vi "source_config.vi"(4 "Multimeter":refnum<visa-resource-name>="GPIB0::7::INSTR", 7 "Sourcemeter":refnum<visa-resource-name>="GPIB0::5::INSTR", 8 "error in (no error)":errorcluster, 9 "Compliance  Level (0.1)":dbl=0.1 step=0.001, 10 "Pas":dbl, 11 "Max":dbl) -> (0 "I(OUT)":dbl[](array[numeric]), 1 "Idd":sgl[](array[numeric]), 2 "error out":errorcluster, 3 "Vdd":dbl[](array[numeric]))   [LabVIEW 2020]
uses:
  2bc7478b-b12c-4ad0-b138-ccb327745d19.vi
  c7dbf4a5-aa7d-4a6e-9432-fd243a290f67.vi
  d3a0e565-199e-45c5-98c3-4e7bd33e65fd.vi
  Keithley 24XX/Public/Data/Read (Single Point).vi
  Keithley 27XX/Keithley 27XX/Public/Data/Read Single Point.vi
  Keithley 24XX/Keithley 24XX.lvlib
  Keithley 27XX/Keithley 27XX/Keithley 27XX.lvlib
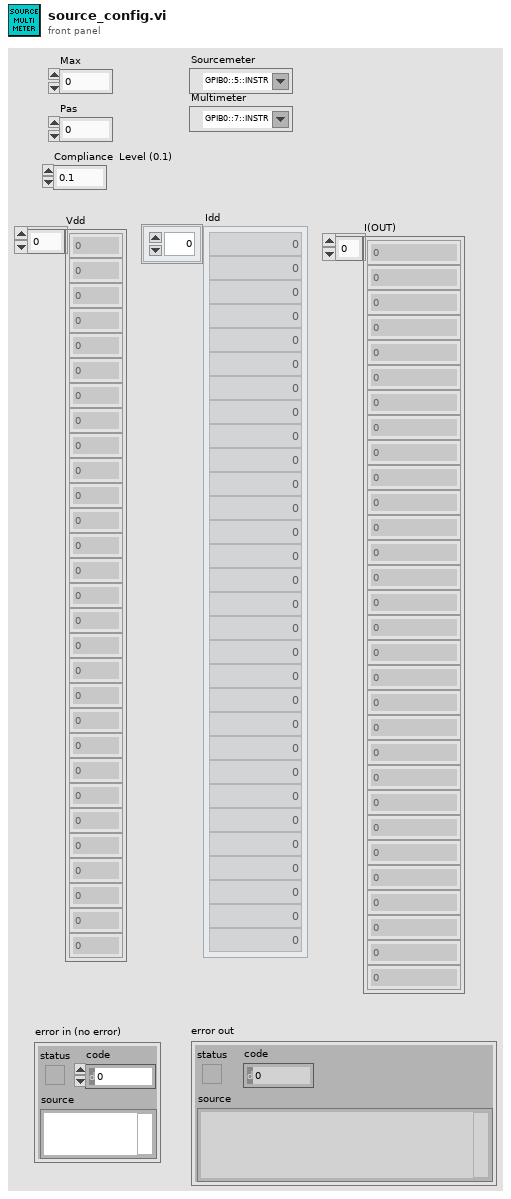
[diagram p1: front panel]
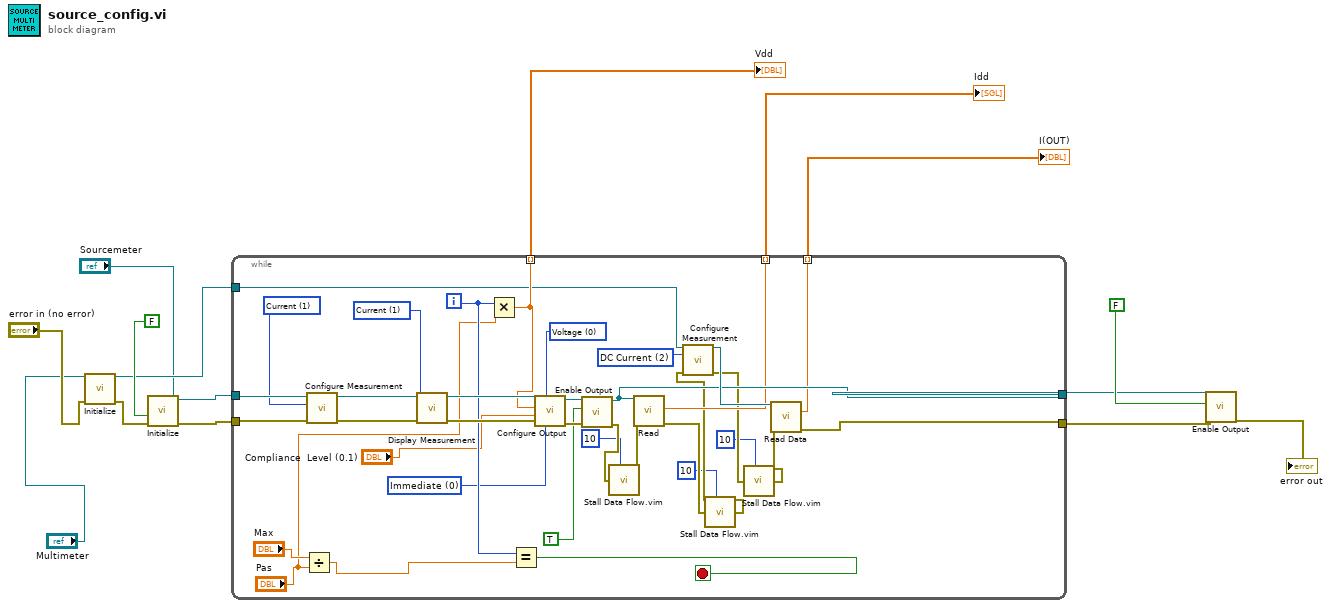
[diagram p0: block diagram]
diagram:
  n1 = call "Initialize.vi"("VISA resource name"="Multimeter", "error in (no error)"="error in (no error)") -> ("VISA resource name out"=w5:refnum<visa-resource-name>, "error out"=w3:errorcluster)  [unwired: 12 in]
  n2 = call "Initialize.vi"("error in (no error)"=w3, "Reset (True)"=FALSE, "VISA resource name"="Sourcemeter") -> ("error out"=w12:errorcluster, "VISA resource name out"=w14:refnum<visa-resource-name>)  [unwired: 7 in]
  n3 = while {
    tunnel: w14 -> [w51]
    tunnel: w12 -> [w50]
    tunnel: [w35] -> w10
    tunnel: [w33] -> w9
    tunnel: [w32] -> w8 mode=indexing
    tunnel: [w31] -> w7 mode=indexing
    tunnel: [w30] -> w6 mode=indexing
    tunnel: w5 -> [w29]
    i -> [w43]
    stop <- w42 stop-if-true
    w34 = u16 0 items=["Voltage", "Current"] ("Source Mode  (0: Voltage)")
    w37 = u16 0 items=["Immediate", "Triggered"] ("Output Type  (0: Immediate)")
    w38 = u16 2 items=["DC Voltage", "AC Voltage", "DC Current", "AC Current", "Resistance", "Four-Wire Resistance", "Temperature", "Frequency", "Period", "Continuity"] ("Function (0: DC Voltage)")
    w46 = u16 1 items=["Voltage", "Current", "Resistance"] ("Displayed Measurement (0: Voltage)")
    w49 = u16 1 items=["Volts", "Current", "Resistance"] ("Function (0: Volts)")
    n4 = Divide(x="Max", y="Pas") -> (x/y=w17:dbl)
    n5 = call "Configure Measurement.vi"("error in (no error)"=w50, "Function (0: Volts)"=w49, "VISA resource name"=w51) -> ("error out"=w47:errorcluster, "VISA resource name out"=w48:refnum<visa-resource-name>)  [unwired: 7 in]
    n6 = call "Display Measurement.vi"("error in (no error)"=w47, "Displayed Measurement (0: Voltage)"=w46, "VISA resource name"=w48) -> ("error out"=w44:errorcluster, "VISA resource name out"=w45:refnum<visa-resource-name>)  [unwired: 7 in]
    n7 = Multiply(x=w43, y="Pas") -> (x*y=w30:dbl)
    n8 = Equal?(x=w43, y=w17) -> (x = y?=w42:bool)
    n9 = call "Configure Output.vi"("Output Type  (0: Immediate)"=w37, "Source Mode  (0: Voltage)"=w34, "error in (no error)"=w44, "Compliance  Level (0.1)"="Compliance  Level (0.1)", "Output Level (0)"=w30, "VISA resource name"=w45) -> ("error out"=w40:errorcluster, "VISA resource name out"=w41:refnum<visa-resource-name>)  [unwired: 4 in]
    n10 = call "Enable Output.vi"("error in (no error)"=w40, "Enable Output (T: Enable)"=TRUE, "VISA resource name"=w41) -> ("error out"=w28:errorcluster, "VISA resource name out"=w33:refnum<visa-resource-name>)  [unwired: 7 in]
    n11 = call "Stall Data Flow.vim"("value in"=w28, "milliseconds to wait"=u32 10) -> ("value out"=w27:errorcluster)  [unwired: 1 out]
    n12 = call-poly "Read.vi"("VISA resource name"=w33, "error in (no error)"=w27) -> ("Current"=w31:sgl, "error out"=w25:errorcluster)  [unwired: 7 in, 5 out]
    n13 = call "Stall Data Flow.vim"("value in"=w25, "milliseconds to wait"=u32 10) -> ("value out"=w24:errorcluster)  [unwired: 1 out]
    n14 = call "Configure Measurement.vi"("VISA resource name"=w29, "Function (0: DC Voltage)"=w38, "error in (no error)"=w24) -> ("VISA resource name out"=w36:refnum<visa-resource-name>, "error out"=w22:errorcluster)  [unwired: 11 in]
    n15 = call "Stall Data Flow.vim"("value in"=w22, "milliseconds to wait"=u32 10) -> ("value out"=w21:errorcluster)  [unwired: 1 out]
    n16 = call-poly "Read Data.vi"("VISA resource name"=w36, "error in (no error)"=w21) -> ("Measurement Data"=w32:dbl, "error out"=w35:errorcluster)  [unwired: 11 in, 1 out]
  }
  "Idd" <- w7
  "I(OUT)" <- w8
  "Vdd" <- w6
  n17 = call "Enable Output.vi"("error in (no error)"=w10, "Enable Output (T: Enable)"=FALSE, "VISA resource name"=w9) -> ("error out"=→"error out":errorcluster)  [unwired: 7 in, 1 out]
